vi "initVariables.vi"   [LabVIEW 2017]
uses:
  globalUtilities.vi
  globalDevices.vi
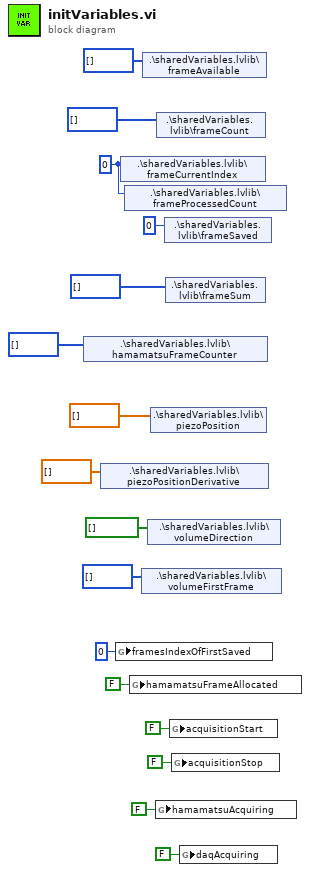
[diagram p0: block diagram]
diagram:
  w2 = 0 ("frameCurrentIndex")
  n1 = shared-variable ".\\sharedVariables.lvlib\\hamamatsuFrameCounter"(u32[] []) -> ()  [unwired: 1 in, 1 out]
  n2 = shared-variable ".\\sharedVariables.lvlib\\piezoPositionDerivative"(dbl[] [] ("piezoPositionDerivative")) -> ()  [unwired: 1 in, 1 out]
  n3 = global write "globalUtilities.vi" "framesIndexOfFirstSaved"(0 ("framesIndexOfFirstSaved")) -> ()
  n4 = shared-variable ".\\sharedVariables.lvlib\\frameCurrentIndex"(w2) -> ()  [unwired: 1 in, 1 out]
  n5 = shared-variable ".\\sharedVariables.lvlib\\frameProcessedCount"(w2) -> ()  [unwired: 1 in, 1 out]
  n6 = global write "globalDevices.vi" "hamamatsuFrameAllocated"(FALSE ("hamamatsuFrameAllocated")) -> ()
  n7 = shared-variable ".\\sharedVariables.lvlib\\volumeFirstFrame"(u32[] [] ("volumeFirstFrame")) -> ()  [unwired: 1 in, 1 out]
  n8 = shared-variable ".\\sharedVariables.lvlib\\frameAvailable"(i32[] [] ("frameAvailable")) -> ()  [unwired: 1 in, 1 out]
  n9 = shared-variable ".\\sharedVariables.lvlib\\volumeDirection"(bool[] [] ("volumeDirection")) -> ()  [unwired: 1 in, 1 out]
  n10 = shared-variable ".\\sharedVariables.lvlib\\piezoPosition"(dbl[] []) -> ()  [unwired: 1 in, 1 out]
  n11 = global write "globalUtilities.vi" "hamamatsuAcquiring"(FALSE ("hamamatsuAcquiring")) -> ()
  n12 = shared-variable ".\\sharedVariables.lvlib\\frameCount"(i32[] []) -> ()  [unwired: 1 in, 1 out]
  n13 = shared-variable ".\\sharedVariables.lvlib\\frameSaved"(u32 0 ("frameSaved")) -> ()  [unwired: 1 in, 1 out]
  n14 = shared-variable ".\\sharedVariables.lvlib\\frameSum"(i64[] []) -> ()  [unwired: 1 in, 1 out]
  n15 = global write "globalUtilities.vi" "acquisitionStart"(FALSE ("acquisitionStart")) -> ()
  n16 = global write "globalUtilities.vi" "acquisitionStop"(FALSE ("acquisitionStop")) -> ()
  n17 = global write "globalUtilities.vi" "daqAcquiring"(FALSE ("daqAcquiring")) -> ()
